vi "KeyValueMap.vi"(8 "error in":errorcluster, 10 "values":string[](array[string])=["\"0.1\"", "\"8008\"", "\" http://localhost\""], 11 "keys":string[](array[string])=["firmwareversion", "port", "url"]) -> (0 "error out":errorcluster, 3 "map out":map{string, string}(c390))   [LabVIEW 2021]
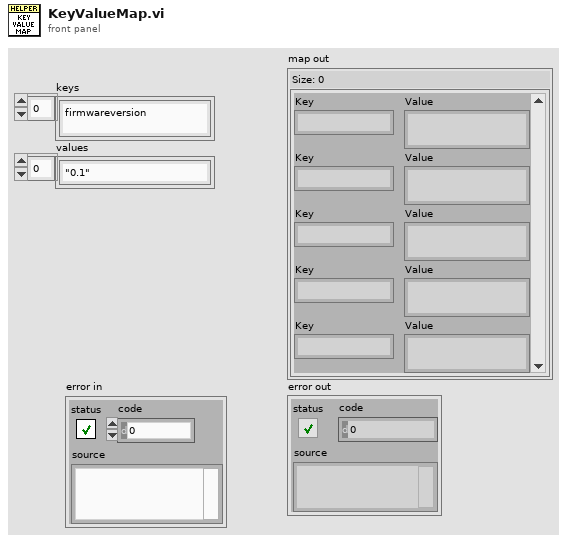
[diagram p1: front panel]
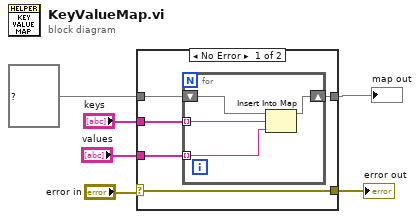
[diagram p0: block diagram]
diagram:
  n1 = case shown="No Error" "error in" {
    selector: "error in" -> [w7 w16]
    tunnel: "keys" -> [w11 _]
    tunnel: "values" -> [w10 _]
    tunnel: map{string, string} {} ("map in") -> [w9 w17]
    tunnel: [w8 w17] -> w3
    tunnel: [w7 w16] -> w1
    frame No Error {
      n2 = for {
        tunnel: w11 -> [w15] mode=indexing
        tunnel: w10 -> [w12] mode=indexing
        shift-right: [w13] -> w8
        shift-left: w9 -> [w14]
        n3 = Insert Into Map(map in=w14, key=w15, value=w12) -> (map out=w13:map{string, string})  [unwired: 2 out]
      }
    }
    frame Error {
    }
  }
  "map out" <- w3
  "error out" <- w1
